vi "OpenLidar.vi"(8 "error in (no error)":errorcluster) -> (0 "error out":errorcluster, 1 "Params Out":cluster{"angle":dbl[], "id":i32[], "kk":dbl[]}, 2 "Measurement Parameters":T1, 3 "VISA Refnum out":refnum<visa-resource-name>)   [LabVIEW 2016]
uses:
  LiDARlib/Type Definitions/Controls/Measurement Parameters.ctl
  LiDARlib/Type Definitions/Controls/Measurement Type.ctl
  <vilib>/imath/engines/lvmath2/RunTimeEngine/Managers/WorkSpace/UID Generator.vi
  <vilib>/imath/engines/lvmath2/RunTimeEngine/BuiltInFunctions/linramp/NIMS_linramp.vi
  <vilib>/imath/engines/lvmath2/RunTimeEngine/IndexRead/NIMS V($).vi
  <instcachedir>/0/NIMS V($)_C593F32C7F6B43C7B1793952E292524F.lvgen/NIMS V($)_C593F32C7F6B43C7B1793952E292524F_001.vi
  <vilib>/imathl/engines/lvmath/Functions/Error Handling/Create Error.vi
  <vilib>/imath/engines/lvmath2/RunTimeEngine/IndexRead/NIMS V(R2).vi
  <instcachedir>/0/NIMS V(R2)_C76619605A0E4E9F8B2FA9389712AC47.lvgen/NIMS V(R2)_C76619605A0E4E9F8B2FA9389712AC47_000.vi
  <vilib>/imath/engines/lvmath2/RunTimeEngine/BuiltInFunctions/mirrorv/NIMS_mirrorv(GColV).vi
  <instcachedir>/0/NIMS_mirrorv(GColV)_C28FB1AB93194ED2915BC859B7BD4827.lvgen/NIMS_mirrorv(GColV)_C28FB1AB93194ED2915BC859B7BD4827_000.vi
  <vilib>/imath/engines/lvmath2/RunTimeEngine/BitwiseOperatorToken/NIMS_Bitwise_Operator_And.vi
  <instcachedir>/0/NIMS_Bitwise_Operator_And_D587B28D2F2E4A5ABF81AE0392B9AD1B.lvgen/NIMS_Bitwise_Operator_And_D587B28D2F2E4A5ABF81AE0392B9AD1B_001.vi
  <vilib>/imath/engines/lvmath2/RunTimeEngine/BitwiseOperatorToken/NIMS_Bitwise_Operator_Or.vi
  <instcachedir>/0/NIMS_Bitwise_Operator_Or_51E58CBCE6004B7AAA420A8AC17D98D6.lvgen/NIMS_Bitwise_Operator_Or_51E58CBCE6004B7AAA420A8AC17D98D6_001.vi
  <vilib>/imath/engines/lvmath2/RunTimeEngine/BuiltInFunctions/findnz/NIMS_[1o]_findnz(GColV).vi
  <instcachedir>/0/NIMS_[1o]_findnz(GColV)_8556557C9365446B906472366DD9B2D8.lvgen/NIMS_[1o]_findnz(GColV)_8556557C9365446B906472366DD9B2D8_000.vi
  <vilib>/imath/engines/lvmath2/RunTimeEngine/ErrorHandling/NIMS_Create Error From Enums.vi
  <vilib>/imath/engines/lvmath2/RunTimeEngine/BuiltInFunctions/numelements/NIMS_numelements.vi
  <instcachedir>/0/NIMS_numelements_A776DA77F73142F68C2F209B523114C5.lvgen/NIMS_numelements_A776DA77F73142F68C2F209B523114C5_004.vi
  <vilib>/imath/engines/lvmath2/RunTimeEngine/RangeToken/NIMS_Range.vi
  <instcachedir>/0/NIMS_Range_A7C094595B484CA7AF10685B02D808ED.lvgen/NIMS_Range_A7C094595B484CA7AF10685B02D808ED_000.vi
  <vilib>/imath/engines/lvmath2/RunTimeSupport/NIMS_Error if Not Equal.vi
  <instcachedir>/0/NIMS_Error if Not Equal_43252A79AD05436189442EC0C5E5AB8A.lvgen/NIMS_Error if Not Equal_43252A79AD05436189442EC0C5E5AB8A_001.vi
  <vilib>/imath/engines/lvmath2/RunTimeEngine/IndexRead/NIMS V(V).vi
  <instcachedir>/0/NIMS V(V)_298D9CB7BFEB42B8BC8D9C3C28AE8C70.lvgen/NIMS V(V)_298D9CB7BFEB42B8BC8D9C3C28AE8C70_000.vi
  <instcachedir>/0/NIMS V(V)_298D9CB7BFEB42B8BC8D9C3C28AE8C70.lvgen/NIMS V(V)_298D9CB7BFEB42B8BC8D9C3C28AE8C70_001.vi
  <vilib>/imath/engines/lvmath2/RunTimeEngine/BuiltInFunctions/mirrorh/NIMS_mirrorh(GRowV).vi
  <instcachedir>/0/NIMS_mirrorh(GRowV)_B6A8CC4EAFBA4F9A82A59460D67BDFF0.lvgen/NIMS_mirrorh(GRowV)_B6A8CC4EAFBA4F9A82A59460D67BDFF0_000.vi
  <vilib>/imath/engines/lvmath2/RunTimeEngine/RunTimeType/NIMS_RunTimeType_From StrictType (excl LVString).vi
  <instcachedir>/0/NIMS_RunTimeType_From StrictType (excl LVString)_BBF44FB49F834B71AF7A14CCEDF8BECD.lvgen/NIMS_RunTimeType_From StrictType (excl LVString)_BBF44FB49F834B71AF7A14CCEDF8BECD_000.vi
  <vilib>/imath/engines/lvmath2/RunTimeEngine/LocalVariableDefStatement/MC_LocalVariableDefStatement_Display.vi
  <vilib>/imath/engines/lvmath2/RunTimeEngine/Managers/SymbolTable/Clear UID.vi
  <vilib>/imath/engines/lvmath2/RunTimeEngine/NodeEndStatement/NIMS_NodeEndStatement_Output.vi
  <instcachedir>/0/NIMS_NodeEndStatement_Output_53EC0D466D134D7ABD903AC30B43404B.lvgen/NIMS_NodeEndStatement_Output_53EC0D466D134D7ABD903AC30B43404B_005.vi
  <instcachedir>/0/NIMS_NodeEndStatement_Output_53EC0D466D134D7ABD903AC30B43404B.lvgen/NIMS_NodeEndStatement_Output_53EC0D466D134D7ABD903AC30B43404B_004.vi
  <vilib>/imath/engines/lvmath2/RunTimeEngine/ErrorHandling/NIMS_Finalize Error.vi
  <vilib>/imath/engines/lvmath2/RunTimeEngine/Managers/SymbolTable/NIMS_WorkSpace.lvlib
panel:
  in  "output cluster":cluster{"angle":dbl[], "id":i32[], "kk":dbl[]}
  in  "VISA Refnum in":refnum<visa-resource-name>="USB0::0x15D1::0x0000::NI-VISA-1002::1::RAW"
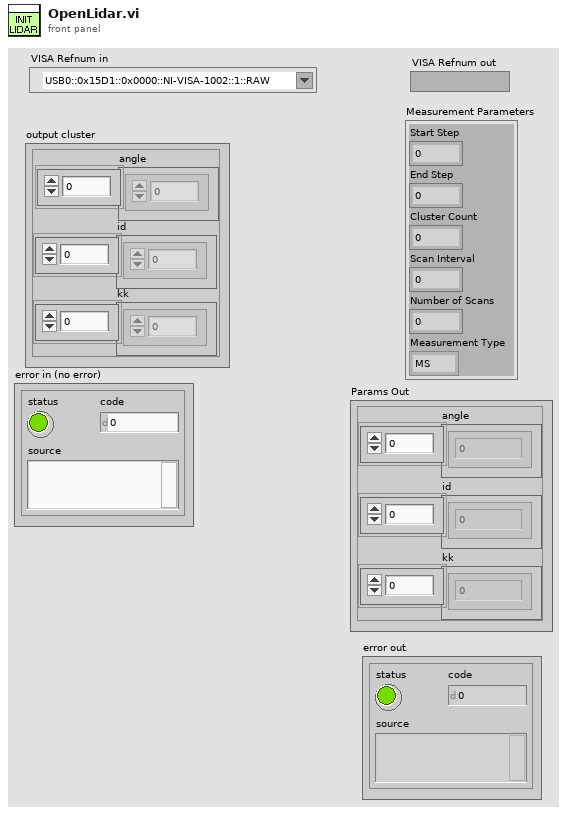
[diagram p1: front panel]
types:
  T1 = typedef "Measurement Parameters.ctl" = cluster{"Start Step":u32, "End Step":u32, "Cluster Count":u32, "Scan Interval":u32, "Number of Scans":u32, "Measurement Type":T2}
  T2 = typedef "Measurement Type.ctl" = enum16{"MS"}
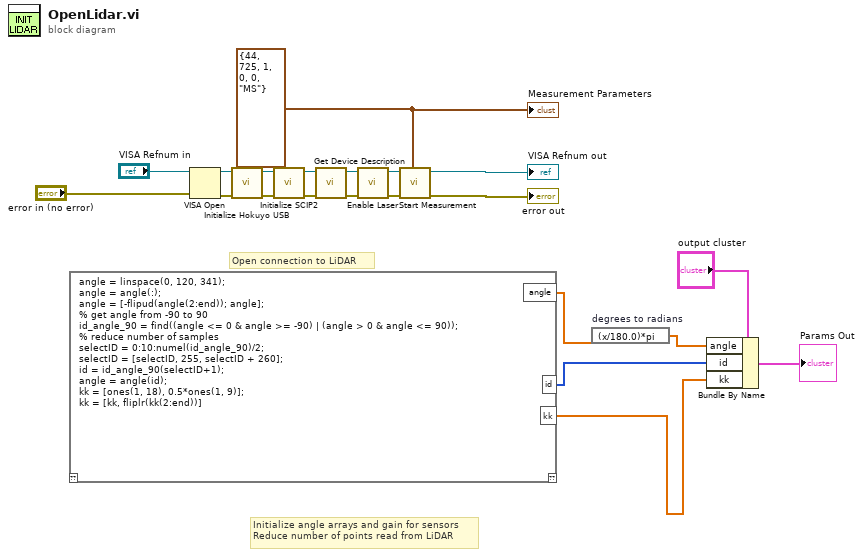
[diagram p0: block diagram]
diagram:
  w19 = T1 {"Start Step"=44, "End Step"=725, "Cluster Count"=1, "Scan Interval"=0, "Number of Scans"=0, "Measurement Type"=enum."MS"} ("Measurement Parameters")
  # "Initialize angle arrays and gain for sensors\nReduce number of points read from LiDAR"
  # "Open connection to LiDAR"
  n1 = mathscript code="angle = linspace(0, 120, 341);\nangle = angle(:);\nangle = [-flipud(angle(2:end)); angle];\n% get angle from -90 to 90\nid_angle_90 = find((angle <= 0 & angle >= -90) | (angle > 0 & angle <= 90));\n% reduce number of samples\nselectID = 0:10:numel(id_angle_90)/2;\nselectID = [selectID, 255, selectID + 260];\nid = id_angle_90(selectID+1);\nangle = angle(id);\nkk = [ones(1, 18), 0.5*ones(1, 9)];\nkk = [kk, fliplr(kk(2:end))]"() -> ("angle"=w3:dbl[], "id"=w7:i32[], "kk"=w6:dbl[])  [unwired: 1 in, 1 out]
  n2 = VISA Open(error in (no error)="error in (no error)", VISA resource name="VISA Refnum in") -> (VISA resource name=w14:refnum<visa-resource-name>, error out=w9:errorcluster)  [unwired: 3 in]
  n3 = call "Initialize Hokuyo USB.vi"("error in (no error)"=w9, "VISA Refnum in"=w14) -> ("error out"=w8:errorcluster, "VISA Refnum out"=w15:refnum<visa-resource-name>)  [unwired: 8 in]
  n4 = call "Initialize SCIP2.vi"("error in (no error)"=w8, "VISA Refnum in"=w15) -> ("error out"=w11:errorcluster, "VISA Refnum out"=w16:refnum<visa-resource-name>)  [unwired: 8 in]
  n5 = call "Get Device Description.vi"("error in (no error)"=w11, "VISA Refnum in"=w16) -> ("error out"=w10:errorcluster, "VISA Refnum out"=w17:refnum<visa-resource-name>)  [unwired: 7 in, 1 out]
  n6 = call "Enable Laser.vi"("error in (no error)"=w10, "VISA Refnum in"=w17) -> ("error out"=w12:errorcluster, "VISA Refnum out"=w18:refnum<visa-resource-name>)  [unwired: 8 in]
  n7 = call "Start Measurement.vi"("error in (no error)"=w12, "Measurement Parameters"=w19, "VISA Refnum in"=w18) -> ("error out"=→"error out":errorcluster, "VISA Refnum out"=→"VISA Refnum out":refnum<visa-resource-name>)  [unwired: 7 in]
  n8 = expression code="(x/180.0)*pi" "degrees to radians"(w3) -> (w2:dbl[])
  n9 = Bundle By Name(cluster="output cluster", "angle"=w2, "id"=w7, "kk"=w6) -> (→"Params Out":cluster{"angle":dbl[], "id":i32[], "kk":dbl[]})
  "Measurement Parameters" <- w19
